vi "Scan Hydra - Cal - Auto.vi"(2 "error in":errorcluster) -> (0 "error out":errorcluster, 1 "next scan":dbl[](array[numeric]) format="%.2f")   [LabVIEW 2019]
uses:
  Global Variables/Global_Variables.vi
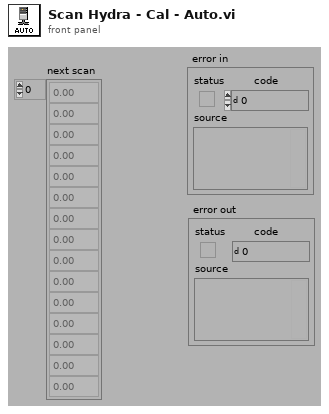
[diagram p1: front panel]
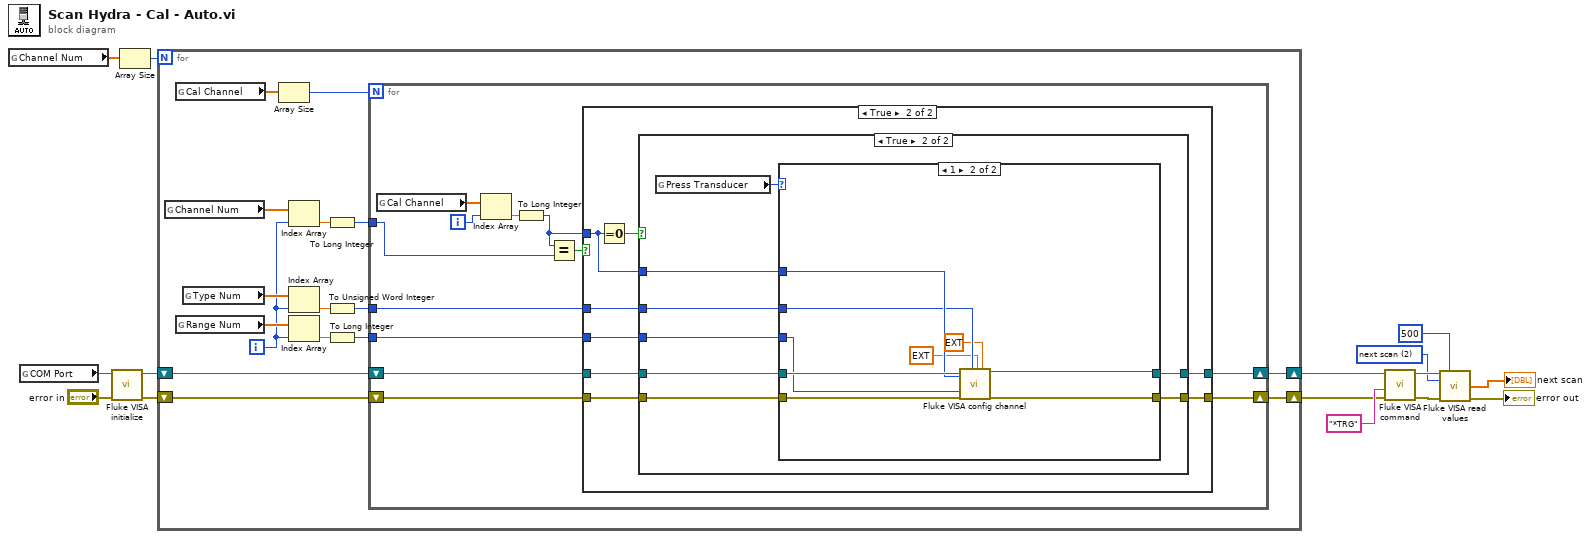
[diagram p0: block diagram]
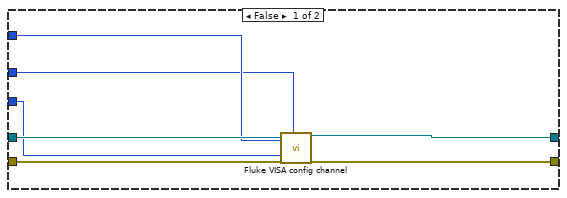
[diagram p3: hidden frame]
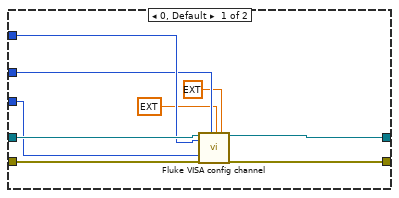
[diagram p4: hidden frame]
diagram:
  w10 = 2 items=["min, max, & last", "monitor value", "next scan", "current total"] ("values to read")
  n1 = global read "Global_Variables.vi" "Channel Num"() -> (w6:dbl[])
  n2 = global read "Global_Variables.vi" "COM Port"() -> (w7:refnum<visa-resource-name>)
  n3 = call "Fluke VISA initialize.vi"("error in (no error)"="error in", "Hydra VISA in"=w7) -> ("error out"=w3:errorcluster, "Hydra VISA out"=w4:refnum<visa-resource-name>)  [unwired: 3 in, 1 out]
  n4 = Array Size(array=w6) -> (size(s)=w5:i32)
  n5 = for {
    N: w5 -> [_]
    shift-right: [w17] -> w1
    shift-left: w4 -> [w23]
    shift-right: [w18] -> w2
    shift-left: w3 -> [w22]
    i -> [w28]
    n6 = global read "Global_Variables.vi" "Channel Num"() -> (w31:dbl[])
    n7 = global read "Global_Variables.vi" "Cal Channel"() -> (w24:dbl[])
    n8 = global read "Global_Variables.vi" "Range Num"() -> (w29:dbl[])
    n9 = global read "Global_Variables.vi" "Type Num"() -> (w30:dbl[])
    n10 = Array Size(array=w24) -> (size(s)=w16:i32)
    n11 = Index Array(array=w31, index=w28) -> (element=w27:dbl)
    n12 = Index Array(array=w30, index=w28) -> (element=w26:dbl)
    n13 = Index Array(array=w29, index=w28) -> (element=w25:dbl)
    n14 = To Long Integer(number=w27) -> (32bit integer=w21:i32)
    n15 = To Unsigned Word Integer(number=w26) -> (unsigned 16bit integer=w20:u16)
    n16 = To Long Integer(number=w25) -> (32bit integer=w19:i32)
    n17 = for {
      N: w16 -> [_]
      tunnel: w21 -> [w40]
      shift-right: [w35] -> w17
      shift-left: w23 -> [w36]
      shift-right: [w34] -> w18
      shift-left: w22 -> [w37]
      tunnel: w20 -> [w32]
      tunnel: w19 -> [w33]
      i -> [w42]
      n18 = global read "Global_Variables.vi" "Cal Channel"() -> (w43:dbl[])
      n19 = Index Array(array=w43, index=w42) -> (element=w41:dbl)
      n20 = To Long Integer(number=w41) -> (32bit integer=w38:i32)
      n21 = Equal?(x=w38, y=w40) -> (x = y?=w39:bool)
      n22 = case shown="True" w39 {
        tunnel: w38 -> [_ w48]
        tunnel: w37 -> [w44 w51]
        tunnel: w36 -> [w45 w52]
        tunnel: [w45 w46] -> w35
        tunnel: [w44 w47] -> w34
        tunnel: w33 -> [_ w50]
        tunnel: w32 -> [_ w49]
        frame False {
        }
        frame True {
          n23 = Equal To 0?(x=w48) -> (x = 0?=w53:bool)
          n24 = case shown="True" w53 {
            tunnel: w52 -> [w59 w67]
            tunnel: w51 -> [w60 w66]
            tunnel: w50 -> [w56 w61]
            tunnel: w49 -> [w57 w62]
            tunnel: w48 -> [w58 w63]
            tunnel: [w55 w65] -> w47
            tunnel: [w54 w64] -> w46
            frame False {
              n25 = call "Fluke VISA config channel.vi"("Hydra VISA in"=w59, "channel"=w58, "range (auto:0)"=w56, "error in (no error)"=w60, "function (off:0)"=w57) -> ("Hydra VISA out"=w54:refnum<visa-resource-name>, "error out"=w55:errorcluster)  [unwired: 13 in]
            }
            frame True {
              n26 = global read "Global_Variables.vi" "Press Transducer"() -> (w68:u16)
              n27 = case shown="1" w68 {
                tunnel: w67 -> [w75 w84]
                tunnel: w66 -> [w77 w86]
                tunnel: [w76 w85] -> w65
                tunnel: [w74 w83] -> w64
                tunnel: w63 -> [w73 w82]
                tunnel: w62 -> [w72 w81]
                tunnel: w61 -> [w71 w80]
                frame 0, Default {
                  n28 = call "Fluke VISA config channel.vi"("Hydra VISA in"=w75, "channel"=w73, "range (auto:0)"=w71, "error in (no error)"=w77, "function (off:0)"=w72, "Mx scaling"=ext 100.0, "+ B scaling"=ext 0.0) -> ("Hydra VISA out"=w74:refnum<visa-resource-name>, "error out"=w76:errorcluster)  [unwired: 11 in]
                }
                frame 1 {
                  n29 = call "Fluke VISA config channel.vi"("Hydra VISA in"=w84, "channel"=w82, "range (auto:0)"=w80, "error in (no error)"=w86, "function (off:0)"=w81, "Mx scaling"=ext 200.0, "+ B scaling"=ext 0.0) -> ("Hydra VISA out"=w83:refnum<visa-resource-name>, "error out"=w85:errorcluster)  [unwired: 11 in]
                }
              }
            }
          }
        }
      }
    }
  }
  n30 = call "Fluke VISA command.vi"("error in (no error)"=w2, "Single Command"="*TRG", "Hydra VISA in"=w1) -> ("error out"=w13:errorcluster, "Hydra VISA out"=w14:refnum<visa-resource-name>)  [unwired: 3 in, 2 out]
  n31 = call "Fluke VISA read values.vi"("Hydra VISA in"=w14, "Byte Count"=u32 500, "values to read"=w10, "error in (no error)"=w13) -> ("next scan"=→"next scan":dbl[], "error out"=→"error out":errorcluster)  [unwired: 4 in, 6 out]
